vi "StripIntersectionGeometry.vi"() -> ()   [LabVIEW 2022 SP3]
uses:
  <vilib>/Platform/NI_3dgraph.lvlib
  <vilib>/Analysis/NI_AALPro.lvlib
  <vilib>/gmath/NI_Gmath.lvlib
panel:
  in  "Case Constant\n(See Context Help) 2":i32=1
  in  "Case Constant\n(See Context Help)":bool
  out "XY Graph":T1(graph)
  out "Output Variable":dbl format="%.2f"
  out "distance":string[](array[string])
  out "in tran zone?":bool
  out "In focal Zone?":bool
  out "Output Cluster":T2 {"r8" format="%.2f"; "r7" format="%.2f"; "r6" format="%.2f"; "r5" format="%.2f"; "r4" format="%.2f"; "r3" format="%.4f"; "r2" format="%.4f"; "r1" format="%.4f"; "r0" format="%.2f"}
  in  "strip":cluster{"radius":dbl, "h":dbl, "w":dbl}={"radius"=10.0, "h"=5.0, "w"=4.0} {"radius" format="%.2f"; "w" format="%.2f"; "h" format="%.2f"}
  in  "P":cluster{"x":dbl, "y":dbl, "z":dbl}={"x"=-4.0, "y"=0.0, "z"=4.0} {"x" format="%.2f"; "z" format="%.2f"; "y" format="%.2f"}
  in  "ct sphere":cluster{"radius":dbl, "theta":dbl, "phi":dbl}={"radius"=10.0, "theta"=160.0, "phi"=100.0} {"radius" format="%.2f"; "phi" format="%.2f"; "theta" format="%.2f"}
  in  "3D Parametric Surface":refnum<k7>(container)
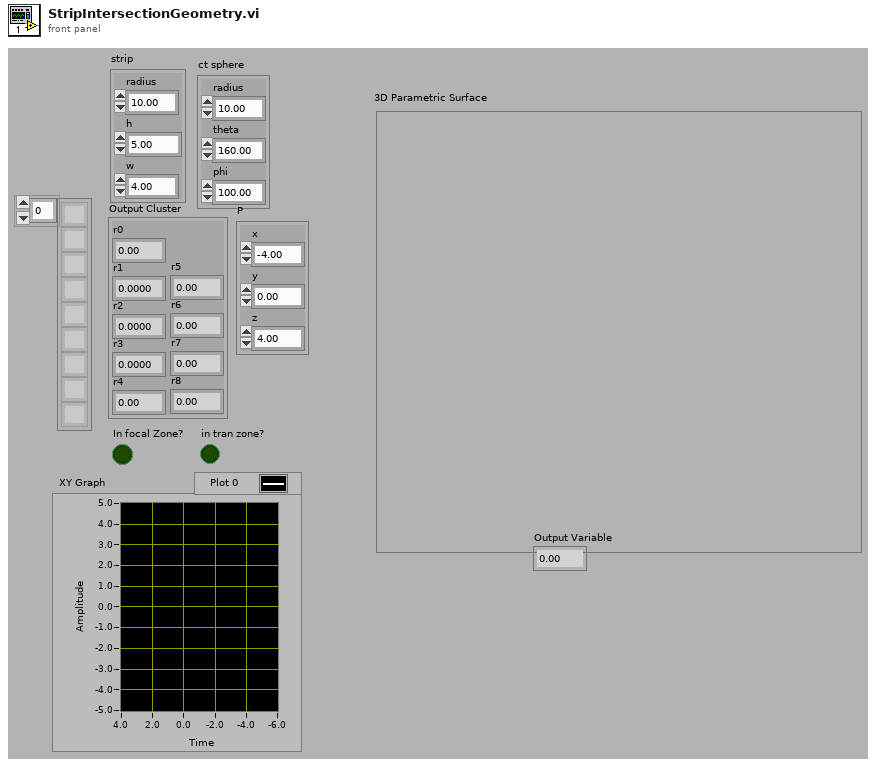
[diagram p1: front panel]
types:
  T1 = cluster{"Array Constant":dbl[], "Array Constant":dbl[]}[]
  T2 = cluster{"r0":dbl, "r1":dbl, "r2":dbl, "r3":dbl, "r4":dbl, "r5":dbl, "r6":dbl, "r7":dbl, "r8":dbl}
  T3 = enum16{"open", "open or create", "create or replace", "create", "open (read only)"}
  T4 = typedef "LVRectTypeDef.ctl" = cluster{"left":i16, "top":i16, "right":i16, "bottom":i16}
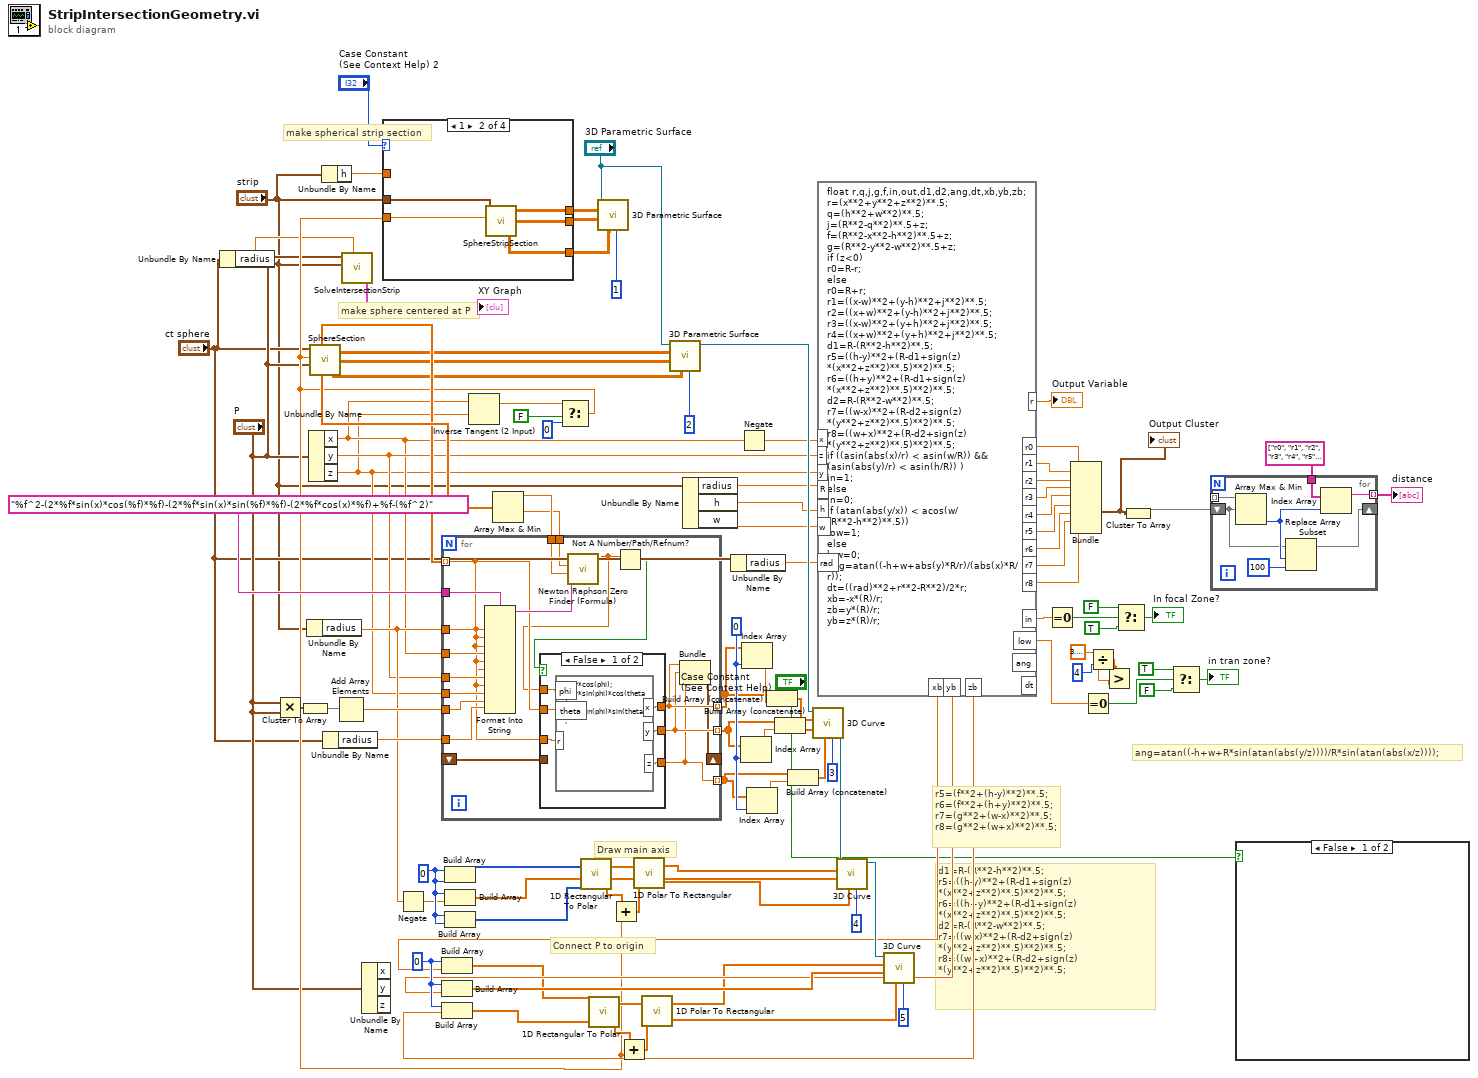
[diagram p0: block diagram]
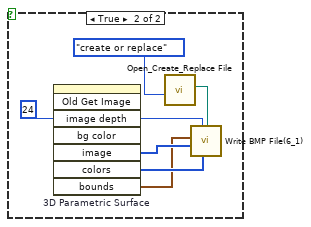
[diagram p2: hidden frame]
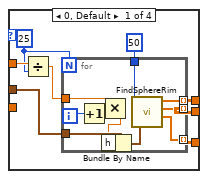
[diagram p3: hidden frame]
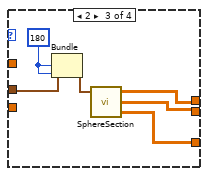
[diagram p4: hidden frame]
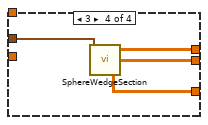
[diagram p5: hidden frame]
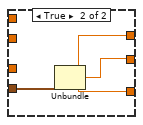
[diagram p6: hidden frame]
diagram:
  w40 = 0
  w89 = 0
  w94 = 0
  # "ang=atan((-h+w+R*sin(atan(abs(y/z))))/R*sin(atan(abs(x/z))));"
  # "d1=R-(R**2-h**2)**.5;\nr5=((h-y)**2+(R-d1+sign(z)\t*(x**2+z**2)**.5)**2)**.5;\nr6=((h+y)**2+(R-d1+sign(z)\t*(x**2+z**2)**.5)**2)**.5;\nd2=R-(R**2-w**2)**.5;\nr7=((w-x)**2+(R-d2+sign(z)\t*(y**2+z**2)**.5)**2)**.5;\nr8=((w+x)**2+(R-d2+sign(z)\t*(y**2+z**2)**.5)**2)**.5;"
  # "r5=(f**2+(h-y)**2)**.5;\nr6=(f**2+(h+y)**2)**.5;\nr7=(g**2+(w-x)**2)**.5;\nr8=(g**2+(w+x)**2)**.5;"
  # "Connect P to origin"
  # "Draw main axis"
  # "make sphere centered at P"
  # "make spherical strip section"
  n1 = Unbundle By Name("ct sphere") -> ("radius"=w6:dbl)
  n2 = Multiply(x="P", y="P") -> (x*y=w101:cluster{"x":dbl, "y":dbl, "z":dbl})
  n3 = Cluster To Array(cluster=w101) -> (array=w100:dbl[])
  n4 = Unbundle By Name("strip") -> ("radius"=w78:dbl)
  n5 = Unbundle By Name("P") -> ("x"=w14:dbl, "y"=w15:dbl, "z"=w13:dbl)
  n6 = Unbundle By Name("strip") -> ("h"=w3:dbl)
  n7 = Unbundle By Name("ct sphere") -> ("radius"=w97:dbl)
  n8 = Add Array Elements(numeric array=w100) -> (sum=w98:dbl)
  n9 = call "SolveIntersectionStrip.vi"("ct"=w6, "strip"="strip", "P"="P") -> ("XY Graph"=→"XY Graph":T1)  [unwired: 1 in, 7 out]
  n10 = Unbundle By Name("P") -> ()  [unwired: 3 out]
  n11 = Negate(x=w78) -> (-x=w90:dbl)
  n12 = Build Array(w94, w94) -> (w28:i32[])
  n13 = Build Array(w94, w90) -> (w92:dbl[])
  n14 = Build Array(w94, w94) -> (w30:i32[])
  n15 = Inverse Tangent (2 Input)(1:w13, 2:w14) -> (0:w12:dbl)
  n16 = Select(t=w12, s=FALSE, f=0) -> (s? t:f=w10:dbl)
  n17 = call "SphereSection.vi"("Ducer"="ct sphere", "Rotate"=w10, "P"="P") -> ("thetas"=w79:dbl[], "phis"=w80:dbl[], "x matrix"=w18:dbl[][], "y matrix"=w17:dbl[][], "z matrix"=w16:dbl[][])  [unwired: 1 out]
  n18 = case shown="1" "Case Constant\n(See Context Help) 2" {
    tunnel: [w111 w127 w133 w137] -> w83
    tunnel: [w110 w126 w132 w136] -> w82
    tunnel: [w109 w125 w131 w135] -> w81
    tunnel: w10 -> [_ w124 _ _]
    tunnel: "strip" -> [w112 w123 w130 w134]
    tunnel: w3 -> [w108 _ _ _]
    frame 0, Default {
      w106 = 25
      n19 = Divide(x=w108, y=w106) -> (x/y=w107:dbl)
      n20 = for {
        N: w106 -> [_]
        tunnel: w112 -> [w115]
        tunnel: [w122] -> w111 mode=indexing
        tunnel: [w121] -> w110 mode=indexing
        tunnel: [w120] -> w109 mode=indexing
        tunnel: w107 -> [w118]
        tunnel: 50 -> [w116]
        i -> [w119]
        n21 = Increment(x=w119) -> (x+1=w117:i32)
        n22 = Multiply(x=w118, y=w117) -> (x*y=w114:dbl)
        n23 = Bundle By Name(cluster=w115, "h"=w114) -> (w113:cluster{"radius":dbl, "h":dbl, "w":dbl})
        n24 = call "FindSphereRim.vi"("number of rim points"=w116, "strip (cm)"=w113) -> ("x"=w122:dbl[], "y"=w121:dbl[], "z"=w120:dbl[])  [unwired: 1 out]
      }
    }
    frame 1 {
      n25 = call "SphereStripSection.vi"("Ducer"=w123, "Rotate"=w124) -> ("x matrix"=w127:dbl[][], "y matrix"=w126:dbl[][], "z matrix"=w125:dbl[][])  [unwired: 4 out]
    }
    frame 2 {
      w128 = 180
      n26 = Bundle(cluster=w130, "h"=w128, "w"=w128) -> (w129:cluster{"radius":dbl, "h":dbl, "w":dbl})  [unwired: 1 out]
      n27 = call "SphereSection.vi"("Ducer"=w129) -> ("x matrix"=w133:dbl[][], "y matrix"=w132:dbl[][], "z matrix"=w131:dbl[][])  [unwired: 2 in, 3 out]
    }
    frame 3 {
      n28 = call "SphereWedgeSection.vi"("Ducer"=w134) -> ("x matrix"=w137:dbl[][], "y matrix"=w136:dbl[][], "z matrix"=w135:dbl[][])  [unwired: 1 in, 4 out]
    }
  }
  n29 = Array Max & Min(array=w80) -> (max value=w85:dbl, min value=w84:dbl)  [unwired: 2 out]
  n30 = for {
    tunnel: "%f^2-(2*%f*sin(x)*cos(%f)*%f)-(2*%f*sin(x)*sin(%f)*%f)-(2*%f*cos(x)*%f)+%f-(%f^2)" ("formula") -> [w148]
    tunnel: w14 -> [w155]
    tunnel: w15 -> [w154]
    tunnel: w78 -> [w146]
    tunnel: w13 -> [w153]
    tunnel: w98 -> [w152]
    tunnel: w97 -> [w151]
    tunnel: w79 -> [w145] mode=indexing
    tunnel: [w143] -> w39 mode=indexing
    tunnel: [w142] -> w37 mode=indexing
    tunnel: [w141] -> w36 mode=indexing
    tunnel: w85 -> [w150]
    tunnel: w84 -> [w149]
    shift-right: [w140] -> _
    shift-left: _ -> [w139]
    n31 = Format Into String(format string=w148, w146, w146, w145, w155, w146, w145, w154, w146, w153, w152, w151) -> (resulting string=w147:string)  [unwired: 2 in, 1 out]
    n32 = call <vilib>:"Newton Raphson Zero Finder (Formula).vi"("formula"=w147, "end"=w150, "start"=w149) -> ("zero"=w138:dbl)  [unwired: 5 in, 3 out]
    n33 = Not A Number/Path/Refnum?(number/path/refnum=w138) -> (NaN/Path/Refnum?=w144:bool)
    n34 = case shown="False" w144 {
      tunnel: [w161 w164] -> w143
      tunnel: [w160 w163] -> w142
      tunnel: [w159 w162] -> w141
      tunnel: w146 -> [w158 _]
      tunnel: w145 -> [w157 _]
      tunnel: w139 -> [_ w165]
      tunnel: w138 -> [w156 _]
      frame False {
        n35 = formula code="z=r*cos(phi);\nx=r*sin(phi)*cos(theta);\ny=r*sin(phi)*sin(theta);"("r"=w158, "phi"=w156, "theta"=w157) -> ("x"=w161:dbl, "y"=w160:dbl, "z"=w159:dbl)
      }
      frame True {
        n36 = Unbundle(w165) -> ("x"=w164:dbl, "y"=w163:dbl, "z"=w162:dbl)
      }
    }
    n37 = Bundle("x"=w143, "y"=w142, "z"=w141) -> (w140:cluster{"x":dbl, "y":dbl, "z":dbl})  [unwired: 1 out]
  }
  n38 = call <vilib>:"1D Rectangular To Polar.vi"("X"=w28, "Y"=w30) -> ("Magnitude"=w26:dbl[], "Phase"=w32:dbl[])  [unwired: 1 out]
  n39 = call <vilib>:"3D Parametric Surface.vi"("plot number (1)"=1, "z matrix"=w81, "y matrix"=w82, "x matrix"=w83, "3D graph"="3D Parametric Surface") -> ()  [unwired: 1 in, 6 out]
  n40 = Add(x=w32, y=w10) -> (x+y=w31:dbl[])
  n41 = call <vilib>:"1D Polar To Rectangular.vi"("Magnitude"=w26, "Phase"=w31) -> ("X"=w27:dbl[], "Y"=w29:dbl[])  [unwired: 1 out]
  n42 = call <vilib>:"3D Parametric Surface.vi"("plot number (1)"=2, "z matrix"=w16, "y matrix"=w17, "x matrix"=w18, "3D graph"="3D Parametric Surface") -> ("3D graph out"=w96:refnum<k7>)  [unwired: 1 in, 5 out]
  n43 = Unbundle By Name("strip") -> ("radius"=w77:dbl, "h"=w76:dbl, "w"=w75:dbl)
  n44 = Unbundle By Name("ct sphere") -> ("radius"=w46:dbl)
  n45 = Negate(x=w14) -> (-x=w65:dbl)
  n46 = Index Array(array=w37, index=w40) -> (element=w38:dbl)
  n47 = Index Array(array=w39, index=w40) -> (element=w42:dbl)
  n48 = Index Array(array=w36, index=w40) -> (element=w41:dbl)
  n49 = Build Array (concatenate)(w39, w42) -> (w44:dbl[])
  n50 = Build Array (concatenate)(w37, w38) -> (w43:dbl[])
  n51 = Build Array (concatenate)(w36, w41) -> (w45:dbl[])
  n52 = call <vilib>:"3D Curve.vi"("plot number (1)"=3, "z vector"=w45, "y vector"=w43, "x vector"=w44, "3D graph"=w96) -> ("3D graph out"=w91:refnum<k7>)  [unwired: 1 in, 5 out]
  n53 = formula code="float r,q,j,g,f,in,out,d1,d2,ang,dt,xb,yb,zb;\nr=(x**2+y**2+z**2)**.5;\nq=(h**2+w**2)**.5;\nj=(R**2-q**2)**.5+z;\nf=(R**2-x**2-h**2)**.5+z;\ng=(R**2-y**2-w**2)**.5+z;\nif (z<0) \nr0=R-r;\nelse\nr0=R+r;\nr1=((x-w)**2+(y-h)**2+j**2)**.5;\nr2=((x+w)**2+(y-h)**2+j**2)**.5;\nr3=((x-w)**2+(y+h)**2+j**2)**.5;\nr4=((x+w)**2+(y+h)**2+j**2)**.5;\nd1=R-(R**2-h**2)**.5;\nr5=((h-y)**2+(R-d1+sign(z)\t*(x**2+z**2)**.5)**2)**.5;\nr6=((h+y)**2+(R-d1+sign(z)\t*(x**2+z**2)**.5)**2)**.5;\nd2=R-(R**2-w**2)**.5;\nr7=((w-x)**2+(R-d2+sign(z)\t*(y**2+z**2)**.5)**2)**.5;\nr8=((w+x)**2+(R-d2+sign(z)\t*(y**2+z**2)**.5)**2)**.5;\nif ((asin(abs(x)/r) < asin(w/R)) &&\n(asin(abs(y)/r) < asin(h/R)) )\nin=1;\nelse\nin=0;\nif (atan(abs(y/x)) < acos(w/(R**2-h**2)**.5))\nlow=1;\nelse\nlow=0;\nang=atan((-h+w+abs(y)*R/r)/(abs(x)*R/r));\ndt=((rad)**2+r**2-R**2)/2*r;\nxb=-x*(R)/r;\nzb=y*(R)/r;\nyb=z*(R)/r;"("y"=w13, "x"=w65, "z"=w15, "R"=w77, "w"=w75, "h"=w76, "rad"=w46) -> ("r0"=w74:dbl, "r1"=w73:dbl, "r2"=w72:dbl, "r3"=w71:dbl, "r4"=w70:dbl, "r5"=w69:dbl, "r6"=w68:dbl, "r7"=w67:dbl, "r8"=w66:dbl, "in"=w63:dbl, "low"=w49:dbl, "r"=→"Output Variable":dbl, "xb"=w35:dbl, "yb"=w34:dbl, "zb"=w33:dbl)  [unwired: 2 out]
  n54 = Build Array(w89, w35) -> (w22:dbl[])
  n55 = Build Array(w89, w34) -> (w87:dbl[])
  n56 = Build Array(w89, w33) -> (w19:dbl[])
  n57 = call <vilib>:"1D Rectangular To Polar.vi"("X"=w22, "Y"=w19) -> ("Magnitude"=w21:dbl[], "Phase"=w25:dbl[])  [unwired: 1 out]
  n58 = Add(x=w25, y=w10) -> (x+y=w24:dbl[])
  n59 = call <vilib>:"1D Polar To Rectangular.vi"("Magnitude"=w21, "Phase"=w24) -> ("X"=w20:dbl[], "Y"=w23:dbl[])  [unwired: 1 out]
  n60 = call <vilib>:"3D Curve.vi"("plot number (1)"=4, "z vector"=w29, "y vector"=w92, "x vector"=w27, "3D graph"=w91) -> ("3D graph out"=w86:refnum<k7>)  [unwired: 1 in, 5 out]
  n61 = call <vilib>:"3D Curve.vi"("plot number (1)"=5, "z vector"=w23, "y vector"=w87, "x vector"=w20, "3D graph"=w86) -> ()  [unwired: 1 in, 6 out]
  n62 = Equal To 0?(x=w63) -> (x = 0?=w62:bool)
  n63 = Bundle("r0"=w74, "r1"=w73, "r2"=w72, "r3"=w71, "r4"=w70, "r5"=w69, "r6"=w68, "r7"=w67, "r8"=w66) -> (w64:T2)  [unwired: 1 out]
  "Output Cluster" <- w64
  n64 = Equal To 0?(x=w49) -> (x = 0?=w48:bool)
  n65 = Divide(x=3.141592653589793, y=4) -> (x/y=w47:dbl)
  n66 = Greater?(x=w47, y=w47) -> ()  [unwired: 1 out]
  n67 = Select(t=FALSE, s=w62, f=TRUE) -> (s? t:f=→"In focal Zone?":bool)
  n68 = Cluster To Array(cluster=w64) -> (array=w53:dbl[])
  n69 = Select(t=TRUE, s=w48, f=FALSE) -> (s? t:f=→"in tran zone?":bool)
  n70 = for {
    tunnel: string[] ["r0", "r1", "r2", "r3", "r4", "r5", "r6", "r7", "r8"] ("Array Constant") -> [w168]
    tunnel: [w171] -> w54 mode=indexing
    shift-right: [w167] -> _
    shift-left: w53 -> [w166]
    tunnel: w53 -> [_] mode=indexing
    n71 = Array Max & Min(array=w166) -> (min index (indices)=w170:i32)  [unwired: 3 out]
    n72 = Replace Array Subset(array=w166, new element=100, index=w170) -> (w167:dbl[])
    n73 = Index Array(array=w168, index=w170) -> (element=w171:string)
  }
  "distance" <- w54
  n74 = case shown="False" "Case Constant\n(See Context Help)" {
    frame False {
    }
    frame True {
      w176 = 24
      n75 = invoke on="3D Parametric Surface" class="AXCont" method="Old Get Image"("image depth"=w176) -> ("image"=w174:u8[], "colors"=w175:u32[], "bounds"=w172:T4)  [unwired: 7 in, 5 out]
      n76 = call <vilib>:"Open_Create_Replace File.vi"("function (open:0)"=T3."create or replace") -> ("new file path"=w173:path)  [unwired: 5 in, 5 out]
      n77 = call <vilib>:"Write BMP File(6_1).vi"("color table"=w175, "depth"=w176, "flattened image data"=w174, "rect"=w172, "path to BMP file"=w173) -> ()  [unwired: 1 in, 6 out]
    }
  }
